vi "Is Valid.vi"(8 "error in (no error)":errorcluster, 11 "Session Handle in":T1) -> (0 "error out":errorcluster, 2 "Valid?":bool, 3 "Session Handle out":T1)   [LabVIEW 2020]
uses:
  Typedefs/Session Handle.ctl
  VariableContainer.lvclass
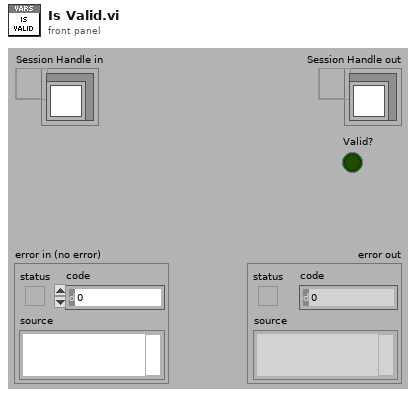
[diagram p1: front panel]
types:
  T1 = typedef "HTS.lvlib/VariableContainer.lvclass/Session Handle.ctl" = refnum<data-value>
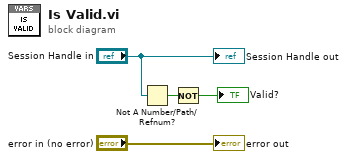
[diagram p0: block diagram]
diagram:
  n1 = Not A Number/Path/Refnum?(number/path/refnum="Session Handle in") -> (NaN/Path/Refnum?=w2:bool)
  n2 = Not(x=w2) -> (.not. x?=→"Valid?":bool)
  "Session Handle out" <- "Session Handle in"
  "error out" <- "error in (no error)"
